vi "wait for recovered modules.vi"(7 "worker pool reference":T2, 8 "error in":errorcluster, 9 "time data in":T1, 10 "run flags in":u8[](array[numeric]), 11 "modules in":T5[](array[typedef])) -> (0 "error out":errorcluster, 2 "run flags out":u8[](array[numeric]), 3 "modules out":T5[](array[typedef]))   [LabVIEW 2013, in "main engine.lvlib"]
doc: "Adds support for reading a module back into the scan after it has recovered from its own error by closing and reinitializing itself."
uses:
  main engine.lvlib
  full module data.ctl
  <vilib>/NI/Tag Bus Module Framework/runtime/TBM module execution interface.lvclass
  module run state.ctl
  async executor/asynchronous executor reference.ctl
  async executor/async message to executor.ctl
  Runtime/async command notification.ctl
  <vilib>/NI/Tag Bus/table/data table.ctl
  Runtime/async error info.ctl
  <vilib>/NI/Tag Bus Module Framework/runtime/error classification.ctl
  <vilib>/NI/Tag Bus Module Framework/module configuration/TBM module configuration.lvclass
  module method data.ctl
  <vilib>/NI/Tag Bus/table/transfer specification.ctl
  <vilib>/NI/Tag Bus/tag/Data Type.ctl
  fault handling spec.ctl
  Configuration/Error Actions.ctl
  worker library/worker comms.ctl
  worker library/worker commands.ctl
  worker library/request fifos.ctl
  worker library/recovery request.ctl
  worker library/rt fault.ctl
  worker library/response fifos.ctl
  worker library/recovery response.ctl
  <vilib>/NI/Module Execution Interface/Engine Runtime/Fault.ctl
  time information.ctl
  worker library/worker pool.lvlib
  <vilib>/NI/Tag Bus/table/data table.lvlib
  <vilib>/NI/Tag Bus/tag/tag descriptor.lvclass
  Configuration/Standard Engine Configuration.lvclass
  <vilib>/NI/Module Execution Interface/Engine Runtime/Engine Runtime Interface.lvclass
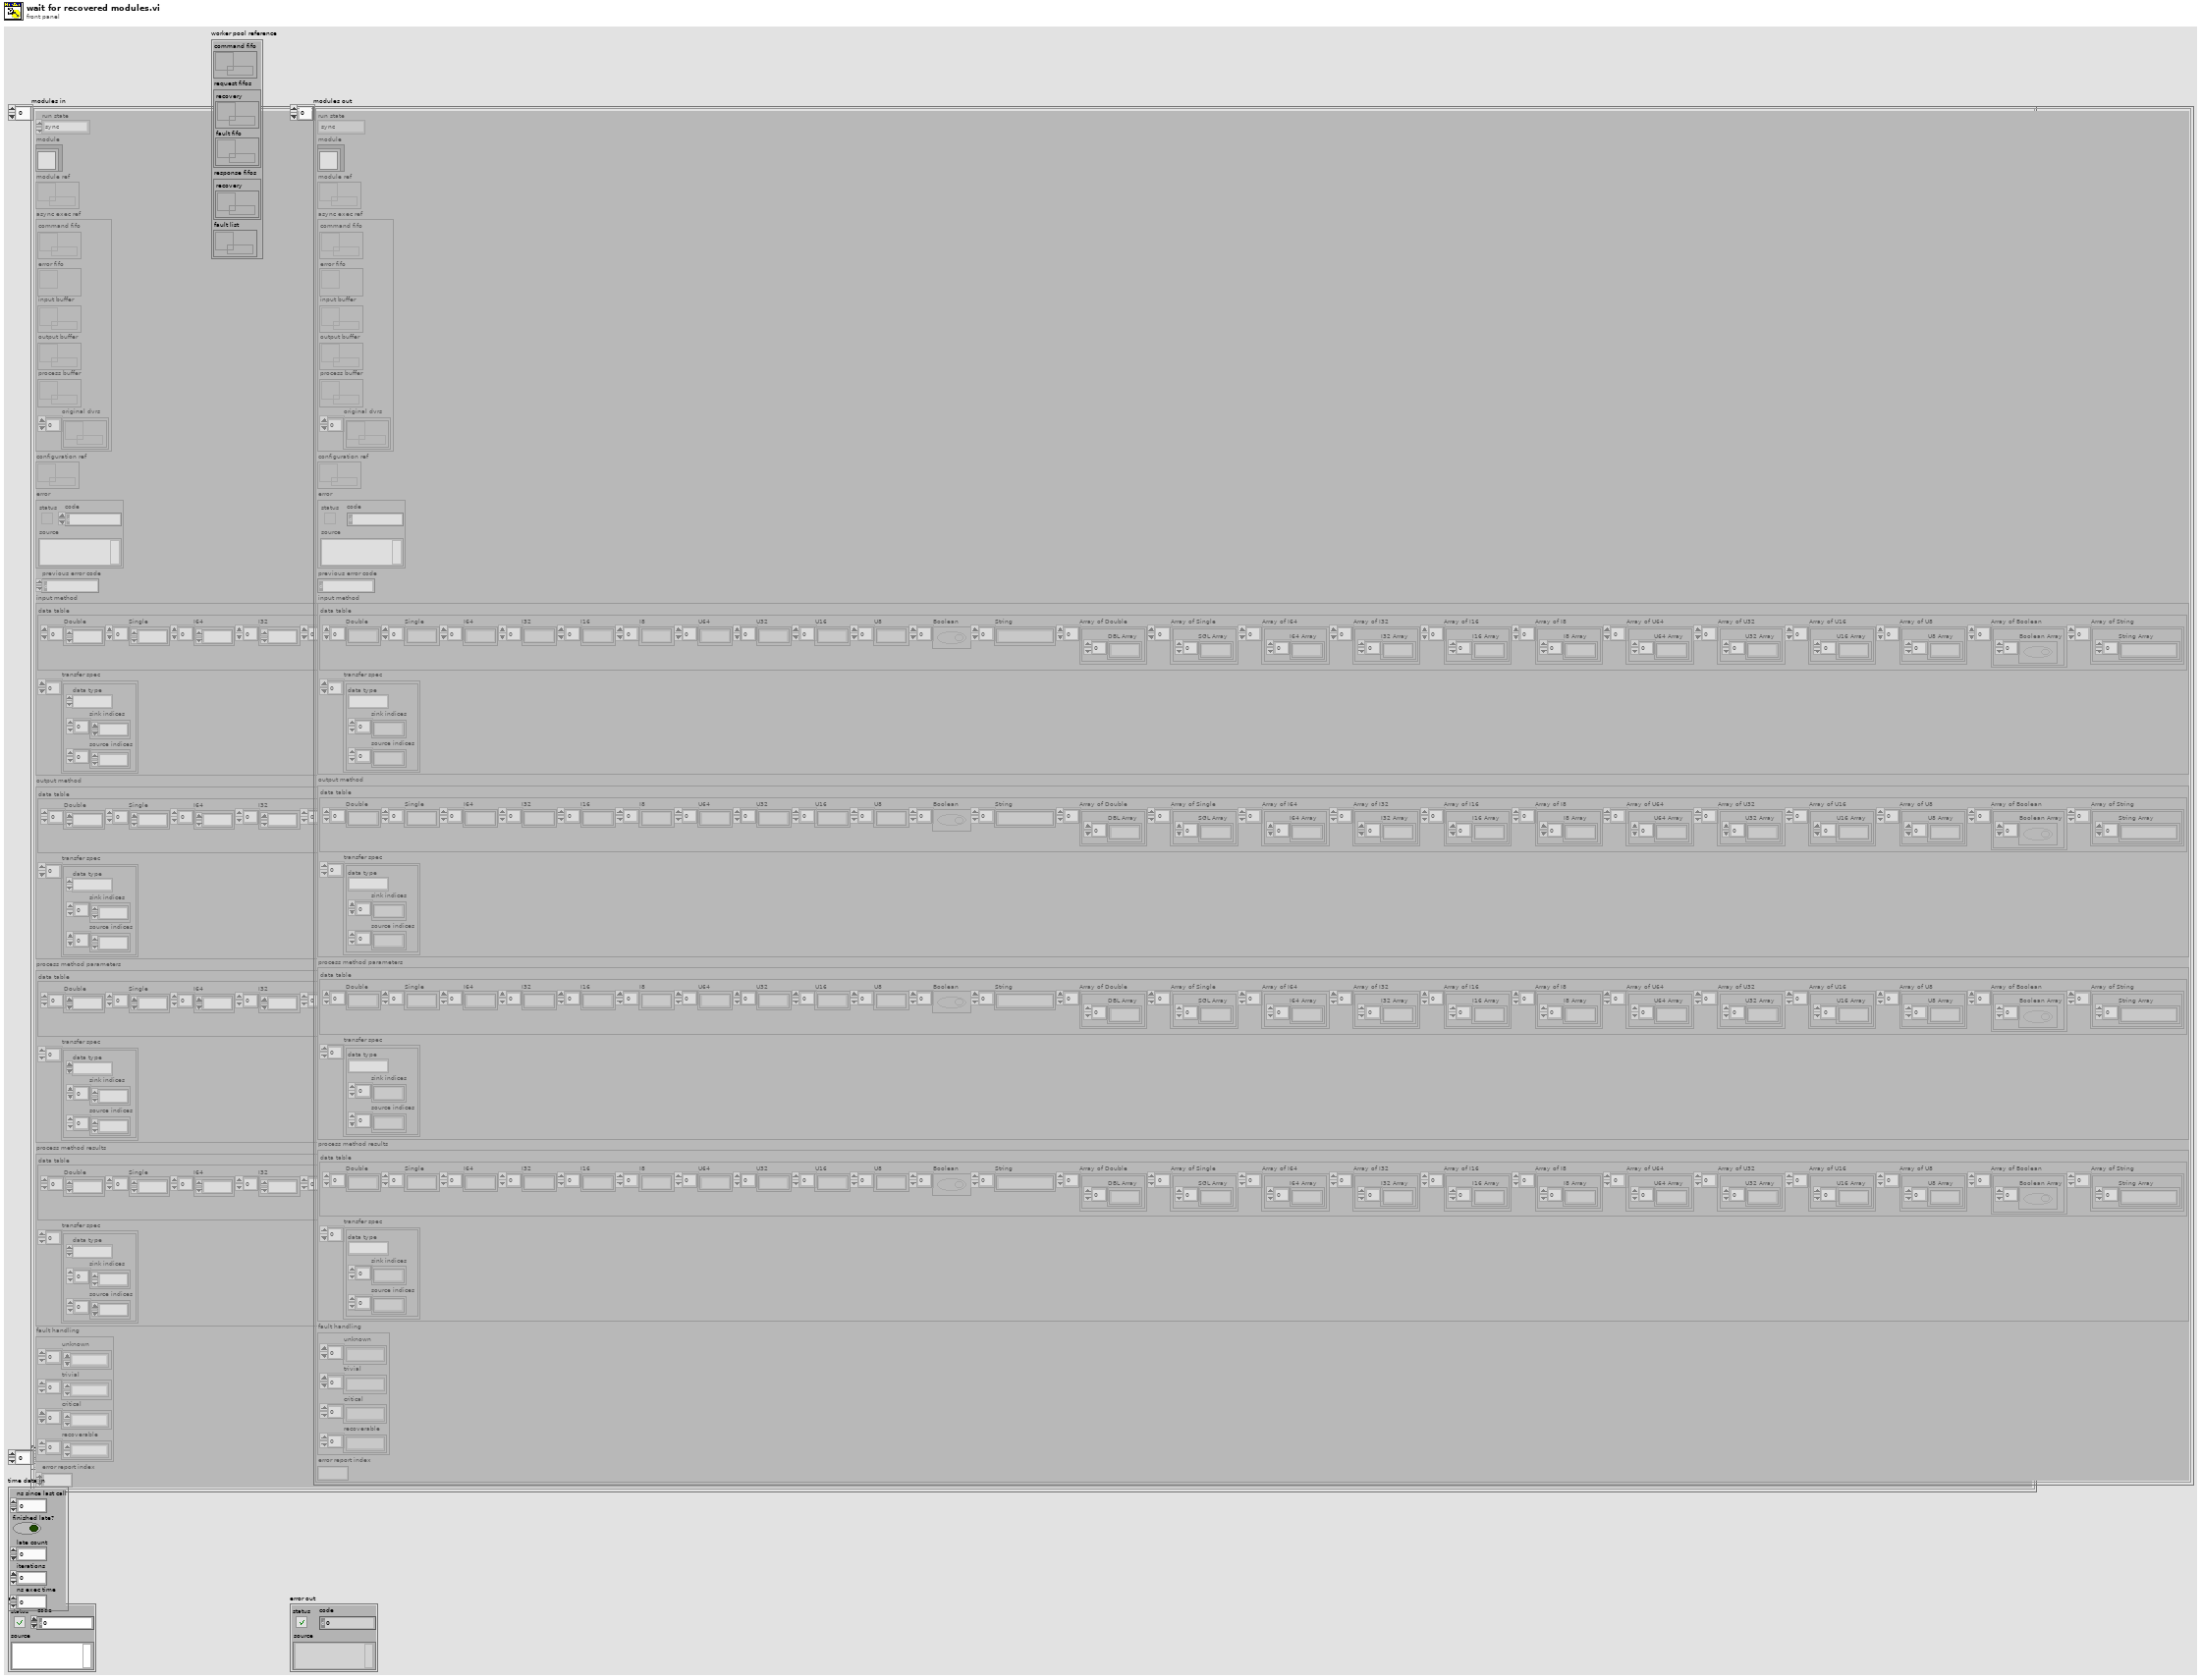
[diagram p1: front panel]
types:
  T1 = typedef "main engine.lvlib/time information.ctl" = cluster{"ns since last call":u64, "finished late?":bool, "late count":u32, "iterations":u64, "ns exec time":u64}
  T2 = typedef "worker pool.lvlib/worker comms.ctl" = cluster{"command fifo":refnum<k33>, "request fifos":T3, "response fifos":T4, "fault list":refnum<data-value>}
  T3 = typedef "worker pool.lvlib/request fifos.ctl" = cluster{"recovery":refnum<k33>, "fault fifo":refnum<k33>}
  T4 = typedef "worker pool.lvlib/response fifos.ctl" = cluster{"recovery":refnum<k33>}
  T5 = typedef "main engine.lvlib/full module data.ctl" = cluster{"run state":T6, "module":refnum<class "TBM module execution interface.lvclass">, "module ref":refnum<data-value>, "async exec ref":T7, "configuration ref":refnum<data-value>, "error":errorcluster, "previous error code":i32, "input method":T8, "output method":T8, "process method parameters":T8, "process method results":T8, "fault handling":T12, "error report index ":i32}
  T6 = typedef "main engine.lvlib/module run state.ctl" = enum16{"sync", "async"}
  T7 = typedef "main engine.lvlib/asynchronous executor reference.ctl" = cluster{"command fifo":refnum<k33>, "error fifo":refnum<k33>, "input buffer":refnum<k33>, "output buffer":refnum<k33>, "process buffer":refnum<k33>, "original dvrs":refnum<data-value>[]}
  T8 = typedef "main engine.lvlib/module method data.ctl" = cluster{"data table":T9, "transfer spec":T10[]}
  T9 = typedef "tag bus.lvlib/data table.lvlib/data table.ctl" = cluster{"Double":dbl[], "Single":sgl[], "I64":i64[], "I32":i32[], "I16":i16[], "I8":i8[], "U64":u64[], "U32":u32[], "U16":u16[], "U8":u8[], "Boolean":bool[], "String":string[], "Array of Double":cluster{"DBL Array":dbl[]}[], "Array of Single":cluster{"SGL Array":sgl[]}[], "Array of I64":cluster{"I64 Array":i64[]}[], "Array of I32":cluster{"I32 Array":i32[]}[], "Array of I16":cluster{"I16 Array":i16[]}[], "Array of I8":cluster{"I8 Array":i8[]}[], "Array of U64":cluster{"U64 Array":u64[]}[], "Array of U32":cluster{"U32 Array":u32[]}[], "Array of U16":cluster{"U16 Array":u16[]}[], "Array of U8":cluster{"U8 Array":u8[]}[], "Array of Boolean":cluster{"Boolean Array":bool[]}[], "Array of String":cluster{"String Array":string[]}[]}
  T10 = typedef "tag bus.lvlib/data table.lvlib/transfer specification.ctl" = cluster{"data type":T11, "sink indices":i32[], "source indices":i32[]}
  T11 = typedef "tag bus.lvlib/tag descriptor.lvclass/Data Type.ctl" = enum16{"Double", "Single", "I64", "I32", "I16", "I8", "U64", "U32", "U16", "U8", "Boolean", "String", "Array of Double", "Array of Single", "Array of I64", "Array of I32", "Array of I16", "Array of I8", "Array of U64", "Array of U32", "Array of U16", "Array of U8", "Array of Boolean", "Array of String"}
  T12 = typedef "main engine.lvlib/fault handling spec.ctl" = cluster{"unknown":T13[], "trivial":T13[], "critical":T13[], "recoverable":T13[]}
  T13 = typedef "Standard Engine Configuration.lvclass/Error Actions.ctl" = enum16{"Clear", "Notify", "Log", "Stop Component", "Stop Engine", "Safe State", "Attempt Recovery"}
  T14 = typedef "worker pool.lvlib/recovery response.ctl" = cluster{"module ref":refnum<data-value>, "engine reference":i32, "original run flags":u8, "success?":bool, "error code":i32}
  T15 = typedef "worker pool.lvlib/recovery request.ctl" = cluster{"module ref":refnum<data-value>, "engine reference":i32, "original run flags":u8, "attempts allowed":u16, "cfg ref":refnum<data-value>}
  T16 = typedef "TBM module execution interface.lvclass/error classification.ctl" = enum16{"unknown", "none", "trivial", "recoverable", "critical"}
  T17 = typedef "worker pool.lvlib/rt fault.ctl" = cluster{"code":i32, "classification":T16, "iteration":u64, "cfg ref":refnum<data-value>}
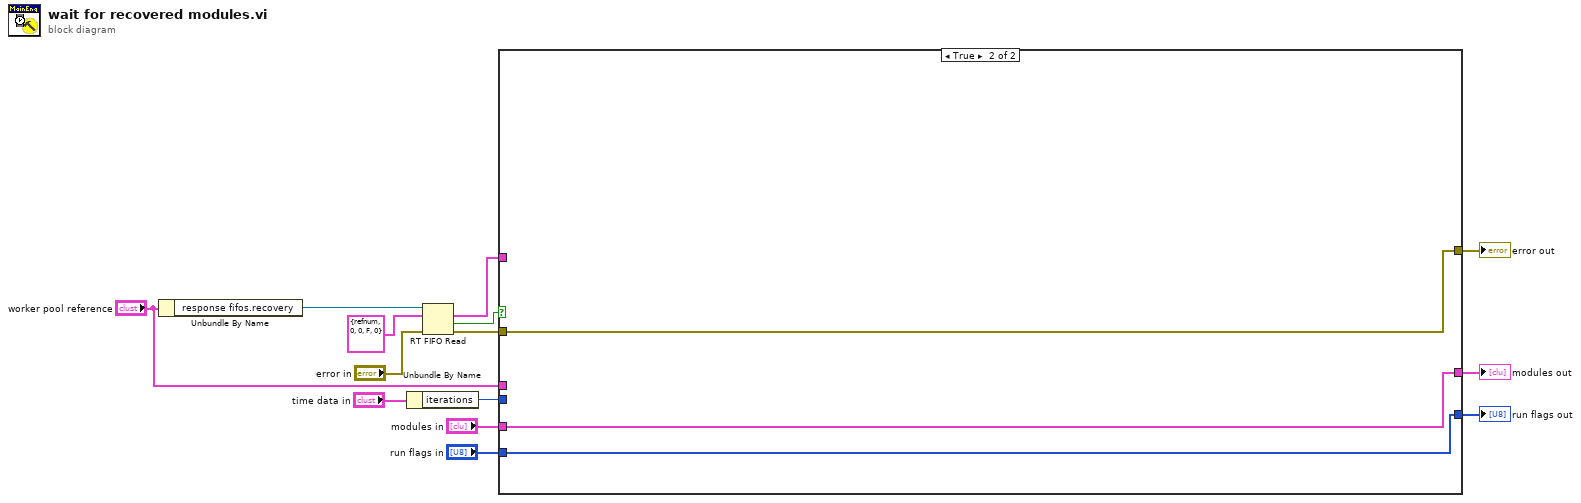
[diagram p0: block diagram]
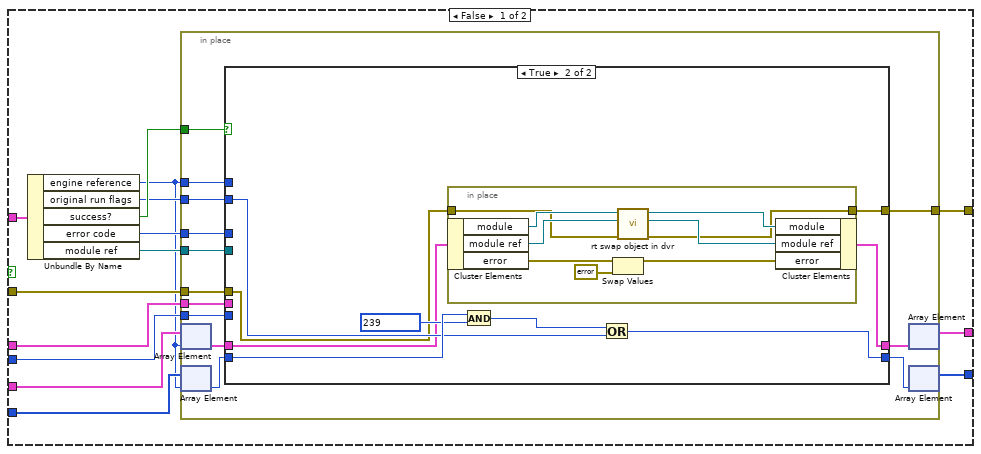
[diagram p2: hidden frame]
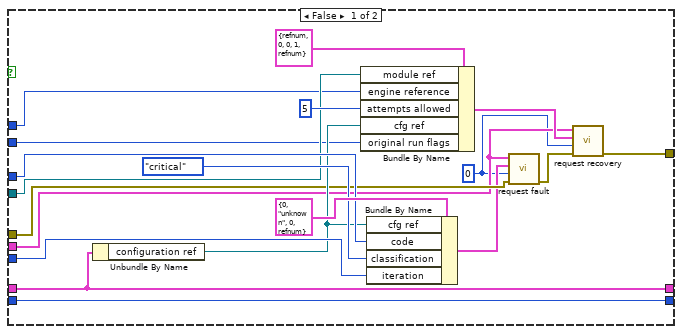
[diagram p3: hidden frame]
diagram:
  n1 = Unbundle By Name("worker pool reference") -> ("response fifos.recovery"=w13:refnum<k33>)
  n2 = Unbundle By Name("time data in") -> ("iterations"=w3:u64)
  n3 = RT FIFO Read(0:w13, 1:T14 {"module ref"=refnum, "engine reference"=0, "original run flags"=0, "success?"=FALSE, "error code"=0} ("element"), 3:"error in") -> (9:w5:T14, 10:w12:bool, 11:w10:errorcluster)  [unwired: 1 in, 2 out]
  n4 = case shown="True" w12 {
    tunnel: [w21 w81] -> w11
    tunnel: w10 -> [w20 w81]
    tunnel: "modules in" -> [w27 w80]
    tunnel: [w24 w80] -> w8
    tunnel: [w25 w79] -> w7
    tunnel: "run flags in" -> [w26 w79]
    tunnel: w5 -> [w28 _]
    tunnel: w3 -> [w18 _]
    tunnel: "worker pool reference" -> [w16 _]
    frame False {
      n5 = Unbundle By Name(w28) -> ("engine reference"=w15:i32, "original run flags"=w22:u8, "success?"=w23:bool, "error code"=w19:i32, "module ref"=w17:refnum<data-value>)
      n6 = in-place {
        in-place-border: w23 -> [w41]
        in-place-border: w22 -> [w34]
        in-place-border: [w36] -> w21
        in-place-border: w20 -> [w35]
        in-place-border: w19 -> [w33]
        in-place-border: w18 -> [w32]
        in-place-border: w17 -> [w31]
        in-place-border: w16 -> [w30]
        in-place-border: w15 -> [w29]
        n7 = in-place-array #1(w27, w15) -> (w39:T5)
        n8 = in-place-array #2(w26, w15) -> (w38:u8)
        n9 = case shown="True" w41 {
          tunnel: [w56 w63] -> w40
          tunnel: w39 -> [w56 w64]
          tunnel: w38 -> [w47 w69]
          tunnel: [w47 w65] -> w37
          tunnel: [w55 w61] -> w36
          tunnel: w35 -> [w45 w62]
          tunnel: w34 -> [w49 w66]
          tunnel: w33 -> [w59 _]
          tunnel: w32 -> [w58 _]
          tunnel: w31 -> [w52 _]
          tunnel: w30 -> [w43 _]
          tunnel: w29 -> [w51 _]
          frame False {
            w42 = 0 ("timeout in ms (0)")
            n10 = Unbundle By Name(w56) -> ("configuration ref"=w50:refnum<data-value>)
            n11 = Bundle By Name(cluster=T15 {"module ref"=refnum, "engine reference"=0, "original run flags"=0, "attempts allowed"=1, "cfg ref"=refnum} ("recovery request"), "module ref"=w52, "engine reference"=w51, "attempts allowed"=u16 5, "cfg ref"=w50, "original run flags"=w49) -> (w48:T15)
            n12 = Bundle By Name(cluster=T17 {"code"=0, "classification"=enum."unknown", "iteration"=0, "cfg ref"=refnum} ("element"), "cfg ref"=w50, "code"=w59, "classification"=error_classification."critical", "iteration"=w58) -> (w44:T17)
            n13 = call "request fault.vi"("error in"=w45, "timeout in ms (0)"=w42, "rt fault"=w44, "worker comms in"=w43) -> ("error out"=w46:errorcluster)  [unwired: 7 in]
            n14 = call "request recovery.vi"("error in"=w46, "timeout in ms (0)"=w42, "recovery request"=w48, "worker comms in"=w43) -> ("error out"=w55:errorcluster)  [unwired: 7 in]
          }
          frame True {
            n15 = in-place {
              in-place-border: w62 -> [w74]
              in-place-border: [w73] -> w61
              n16 = in-place-cluster #3(w64) -> ("module"=w78:refnum<class "TBM module execution interface.lvclass">, "module ref"=w75:refnum<data-value>, "error"=w72:errorcluster)
              n17 = Swap Values(12:w72, 14:errorcluster {"status"=FALSE, "code"=0, "source"=""} ("error")) -> (1:w71:errorcluster)  [unwired: 1 in, 1 out]
              n18 = call "rt swap object in dvr.vi"("error in"=w74, "module ref in in"=w75, "module in"=w78) -> ("error out"=w73:errorcluster, "module ref out"=w76:refnum<data-value>, "module out"=w77:refnum<class "TBM module execution interface.lvclass">)  [unwired: 6 in]
              n19 = in-place-cluster #3("module"=w77, "module ref"=w76, "error"=w71) -> (w63:T5)
            }
            n20 = And(x=w69, y=u8 239) -> (x .and. y?=w67:u8)
            n21 = Or(x=w67, y=w66) -> (x .or. y?=w65:u8)
          }
        }
        n22 = in-place-array #1(w40) -> (w24:T5[])  [unwired: 1 out]
        n23 = in-place-array #2(w37) -> (w25:u8[])  [unwired: 1 out]
      }
    }
    frame True {
    }
  }
  "error out" <- w11
  "run flags out" <- w7
  "modules out" <- w8
